vi "Write Subpanel Refnum.vi"(7 "Force Overwrite? (F)":bool, 8 "error in (no error)":errorcluster, 10 "SubPnl Refnum":refnum<vi>, 11 "IViewModel In":refnum<class "IViewModel.lvclass">) -> (0 "error out":errorcluster, 3 "IViewModel Out":refnum<class "IViewModel.lvclass">)   [LabVIEW 2015, in "IViewModel.lvlib" / "IViewModel.lvclass"]
doc: "<License>\nCopyright © 2017 Composed Systems, LLC | All rights reserved\nwww.composed.io\n\nAuthor: Ethan Stern <ethan.stern@composed.io>\n\nThis software is provided \"AS IS\" WITHOUT WARRANTIES, either express or implied, AND IS FOR EDUCATIONAL PURPOSES ONLY.\n</License>"
uses:
  IViewModel.lvclass
  IViewModel.lvclass/IViewModel.ctl
  <vilib>/Composed Systems/Protected Subpanel/ProtectedSubpanel.lvclass
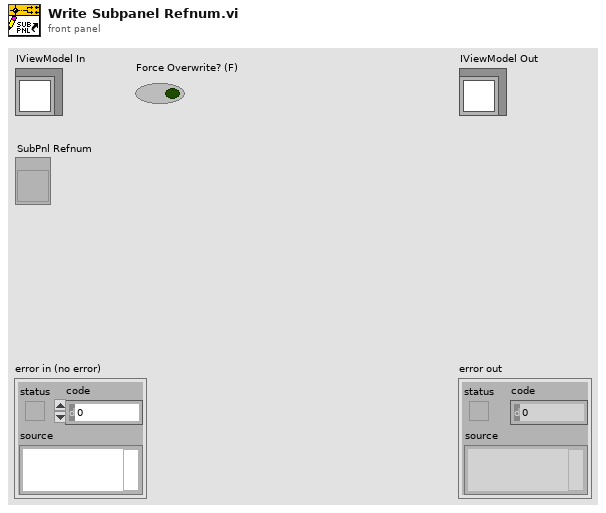
[diagram p1: front panel]
types:
  T1 = typedef "ProtectedSubpanel.lvlib/ProtectedSubpanel.lvclass/Protected Subpanel Reference.ctl" = refnum<data-value>
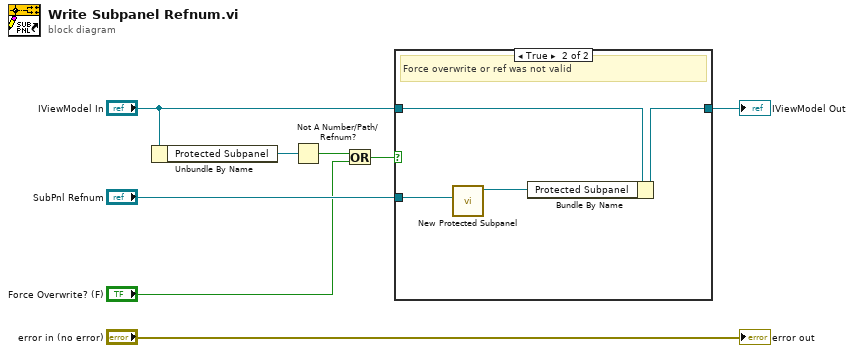
[diagram p0: block diagram]
diagram:
  n1 = Unbundle By Name("IViewModel In") -> ("Protected Subpanel"=w5:T1)
  n2 = Not A Number/Path/Refnum?(number/path/refnum=w5) -> (NaN/Path/Refnum?=w4:bool)
  n3 = Or(x=w4, y="Force Overwrite? (F)") -> (x .or. y?=w1:bool)
  n4 = case shown="True" w1 {
    tunnel: [w9 w13] -> w7
    tunnel: "SubPnl Refnum" -> [_ w11]
    tunnel: "IViewModel In" -> [w9 w12]
    frame False {
      # "Keep pre-existing refnum"
    }
    frame True {
      # "Force overwrite or ref was not valid"
      n5 = call <vilib>:"New Protected Subpanel.vi"("SubPnl Refnum"=w11) -> ("Protected Subpanel"=w10:T1)  [unwired: 9 in, 1 out]
      n6 = Bundle By Name(cluster=w12, "Protected Subpanel"=w10) -> (w13:refnum<class "IViewModel.lvclass">)
    }
  }
  "IViewModel Out" <- w7
  "error out" <- "error in (no error)"
